vi "onecycle.vi"(3 "rotate orientation":string(combo)="clockwise", 4 "task/channels in trotate orientation":refnum<k21>="orientationPort2", 5 "steeper Motor Speed":u32(knob)=25 scale=20.0..100.0, 6 "no Of Step":i32, 7 "task/channels in toggle (step)":refnum<k21>="port01enable") -> (0 "Numeric":i32, 1 "number of samples written":u32, 2 "number of samples written 3":u32)   [LabVIEW 2016]
uses:
  <vilib>/DAQmx/write.llb/DAQmx Write (Digital 1D Bool NChan 1Samp 1Line).vi
  <vilib>/DAQmx/write.llb/DAQmx Write (Digital Bool 1Line 1Point).vi
  <vilib>/DAQmx/miscellaneous.llb/DAQmx Fill In Error Info.vi
panel:
  in  "stepperMotor_Control":enum32{"settingPort", "settingMotor", "view"}(tab)
  out "number of samples written 2":u32
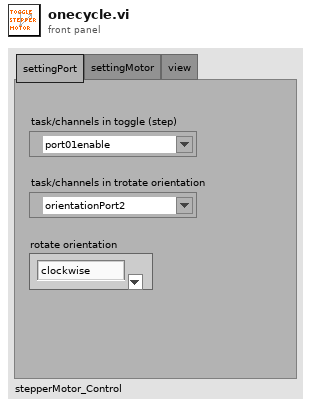
[diagram p1: front panel]
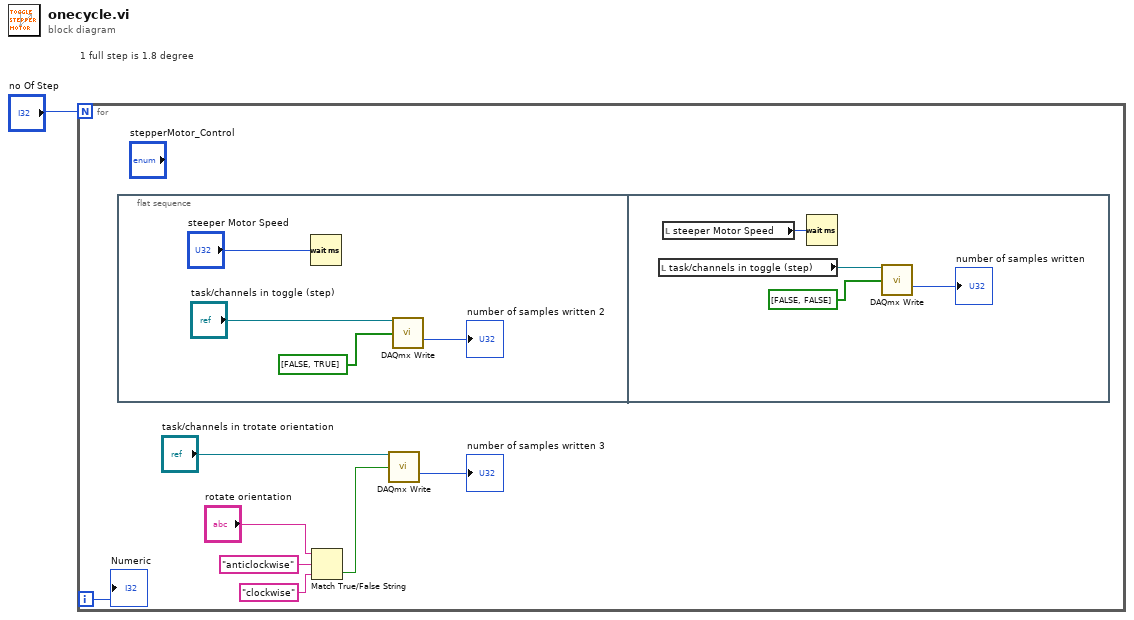
[diagram p0: block diagram]
diagram:
  # "1 full step is 1.8 degree"
  n1 = for {
    N: "no Of Step" -> [_]
    i -> [w2]
    n2 = flat-sequence {
      frame #0 {
        n3 = Wait (ms)(milliseconds to wait="steeper Motor Speed") -> ()  [unwired: 1 out]
        n4 = call-poly <vilib>:"DAQmx Write.vi"("task/channels in"="task/channels in toggle (step)", "data"=bool[] [FALSE, TRUE]) -> ("number of samples written per channel"=→"number of samples written 2":u32)  [unwired: 11 in, 2 out]
      }
      frame #1 {
        n5 = local read "task/channels in toggle (step)"() -> (w13:refnum<k21>)
        n6 = local read "steeper Motor Speed"() -> (w14:u32)
        n7 = Wait (ms)(milliseconds to wait=w14) -> ()  [unwired: 1 out]
        n8 = call-poly <vilib>:"DAQmx Write.vi"("task/channels in"=w13, "data"=bool[] [FALSE, FALSE]) -> ("number of samples written per channel"=→"number of samples written":u32)  [unwired: 11 in, 2 out]
      }
    }
    n9 = Match True/False String(2:"clockwise" ("false string"), 3:"anticlockwise" ("true string"), 4:"rotate orientation") -> (0:w4:bool)  [unwired: 1 out]
    n10 = call-poly <vilib>:"DAQmx Write.vi"("task/channels in"="task/channels in trotate orientation", "data"=w4) -> ("number of samples written per channel"=→"number of samples written 3":u32)  [unwired: 11 in, 2 out]
    "Numeric" <- w2
  }
